vi "NotifyIcon Set.vi"(8 "error in (no error)":errorcluster, 9 "Icon Name":string, 10 "Icon path":path, 11 "Model in":refnum<class "Model.lvclass">) -> (0 "error out":errorcluster, 3 "Model out":refnum<class "Model.lvclass">)   [LabVIEW 2021, in "Model.lvlib" / "Model.lvclass"]
uses:
  Model.lvclass
  Model.lvclass/Model.ctl
  <vilib>/Averna/Notify Icon/NotifyIcon.llb/GetSelectedItemEvent.vi
  <vilib>/Averna/Notify Icon/NotifyIcon.llb/SetVisible.vi
  <vilib>/Averna/Notify Icon/NotifyIcon.llb/SetMenuDefaultItem.vi
  <vilib>/Averna/Notify Icon/NotifyIcon.llb/SetTipText.vi
  <vilib>/Averna/Notify Icon/NotifyIcon.llb/NotifyIcon.lvclass
  <userlib>/John_Lib/TopPath/TopPath.lvlib
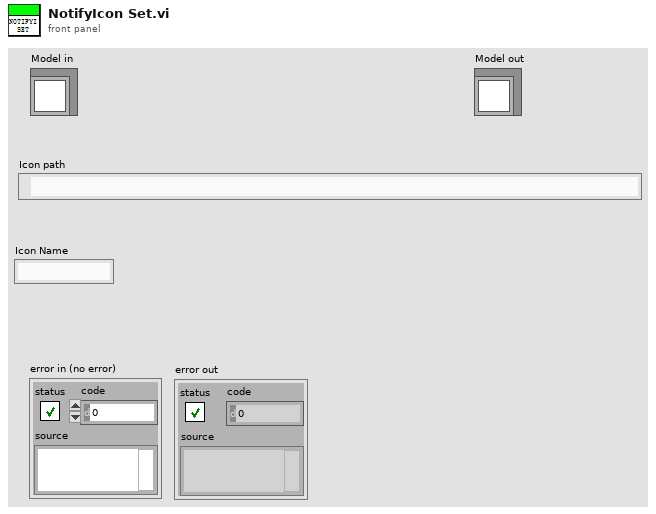
[diagram p1: front panel]
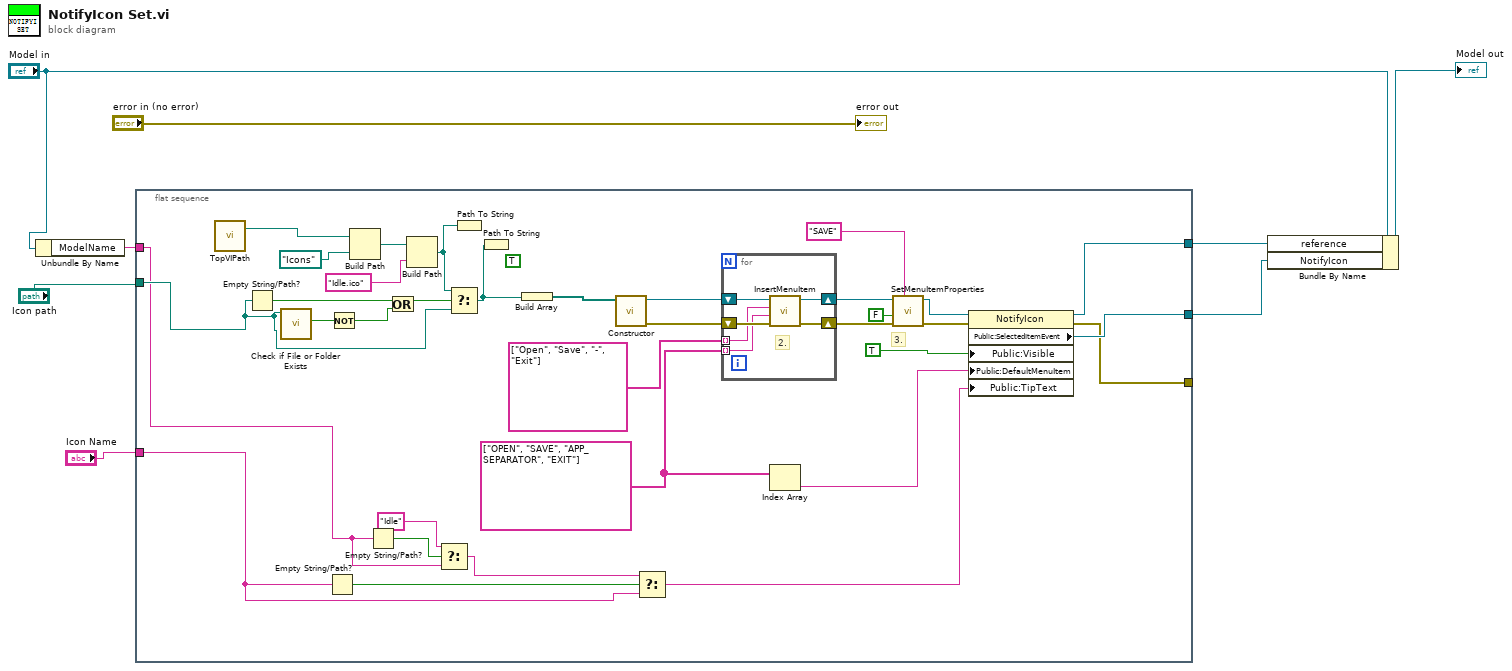
[diagram p0: block diagram]
diagram:
  n1 = Unbundle By Name("Model in") -> ("ModelName"=w1:string)
  n2 = flat-sequence {
    tunnel: [w20] -> w3
    tunnel: [w19] -> _
    tunnel: "Icon Name" -> [w16]
    tunnel: "Icon path" -> [w15]
    tunnel: [w14] -> w4
    tunnel: w1 -> [w11]
    frame #0 {
      (unwired) TRUE ("DisplayDialog")
      w26 = string[] ["OPEN", "SAVE", "APP_SEPARATOR", "EXIT"]
      # "3."
      n3 = call <userlib>:"TopVIPath.vi"() -> ("ConfigFile path"=w35:path)  [unwired: 1 in, 2 out]
      n4 = Empty String/Path?(string/path=w15) -> (empty?=w36:bool)
      n5 = call <vilib>:"Check if File or Folder Exists.vi"("path"=w15) -> ("file or folder exists?"=w41:bool)  [unwired: 8 in, 2 out]
      n6 = Empty String/Path?(string/path=w16) -> (empty?=w13:bool)
      n7 = Not(x=w41) -> (.not. x?=w42:bool)
      n8 = Build Path(base path=w35, name or relative path=path "Icons") -> (appended path=w37:path)
      n9 = Empty String/Path?(string/path=w11) -> (empty?=w12:bool)
      n10 = Or(x=w36, y=w42) -> (x .or. y?=w40:bool)
      n11 = Build Path(base path=w37, name or relative path="Idle.ico") -> (appended path=w18:path)
      n12 = Select(t="Idle", s=w12, f=w11) -> (s? t:f=w9:string)
      n13 = Select(t=w18, s=w40, f=w15) -> (s? t:f=w17:path)
      n14 = Path To String(path=w18) -> ()  [unwired: 1 out]
      n15 = Path To String(path=w17) -> ()  [unwired: 1 out]
      n16 = Build Array(w17) -> (w34:path[])
      n17 = call <vilib>:"Constructor.vi"("IconFilePathList"=w34) -> ("error out"=w22:errorcluster, "NotifyIcon"=w23:refnum<class "NotifyIcon.lvclass">)  [unwired: 9 in]
      n18 = Select(t=w9, s=w13, f=w16) -> (s? t:f=w21:string)
      n19 = for {
        shift-right: [w47] -> w32
        shift-left: w22 -> [w48]
        tunnel: string[] ["Open", "Save", "-", "Exit"] -> [w46] mode=indexing
        tunnel: w26 -> [w45] mode=indexing
        shift-right: [w43] -> w29
        shift-left: w23 -> [w44]
        # "2."
        n20 = call <vilib>:"InsertMenuItem.vi"("error in"=w48, "ItemTag"=w45, "ItemName"=w46, "NotifyIcon in"=w44) -> ("error out"=w47:errorcluster, "NotifyIcon out"=w43:refnum<class "NotifyIcon.lvclass">)  [unwired: 6 in]
      }
      n21 = Index Array(array=w26) -> (element=w33:string)  [unwired: 1 in]
      n22 = call <vilib>:"SetMenuItemProperties.vi"("ItemTag"="SAVE", "error in"=w32, "Enabled"=FALSE, "NotifyIcon in"=w29) -> ("error out"=w31:errorcluster, "NotifyIcon out"=w30:refnum<class "NotifyIcon.lvclass">)  [unwired: 6 in]
      n23 = property class="NotifyIcon"(reference=w30, error in=w31, "Public:Visible"=TRUE ("Visible"), "Public:DefaultMenuItem"=w33, "Public:TipText"=w21) -> (reference out=w14:refnum<class "NotifyIcon.lvclass">, error out=w19:errorcluster, "Public:SelectedItemEvent"=w20:refnum<user-event>)
    }
  }
  n24 = Bundle By Name(cluster="Model in", "reference"=w4, "NotifyIcon"=w3) -> (→"Model out":refnum<class "Model.lvclass">)
  "error out" <- "error in (no error)"
